vi "Dispose Gabor RefNum.vi"(5 "error in (no error)":errorcluster, 8 "RefNum in":T1) -> (0 "error out":errorcluster)   [LabVIEW 2017, in "SoundVib_Gabor.lvlib"]
doc: "Disposes of the data block referenced by <B>RefNum in</B>."
uses:
  <vilib>/addons/Sound and Vibration/Order Analysis/Gabor Order Tracking/SoundVib_Gabor.lvlib
  <vilib>/addons/Sound and Vibration/Order Analysis/Ref Gabor Order Tracking/GT RefNum.ctl
  <resource>/sndvib.dll
panel:
  # "Dispose Gabor RefNum"
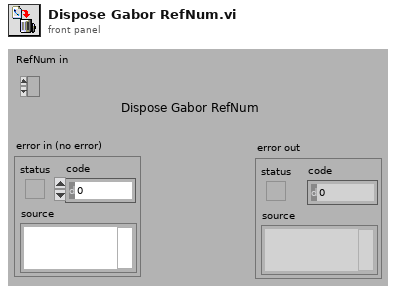
[diagram p1: front panel]
types:
  T1 = typedef "SoundVib_Gabor.lvlib/GT RefNum.ctl" = refnum<k1>
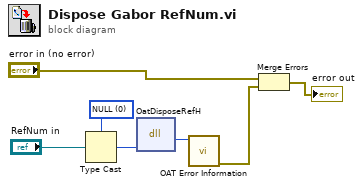
[diagram p0: block diagram]
diagram:
  w4 = u32 0 items=["NULL"]
  n1 = Type Cast(type=w4, x="RefNum in") -> (*(type *) &x=w6:u32)
  n2 = dll-call lib="C:/Program Files (x86)/National Instruments/LabVIEW 2017/resource/sndvib.*" fn="OatDisposeRefH"("Ref In"=w6) -> ("return type"=w7:i32)  [unwired: 4 in, 2 out]
  n3 = call <vilib>:"OAT Error Information.vi"("error code"=w7) -> ("error out"=w1:errorcluster)  [unwired: 6 in]
  n4 = Merge Errors("error in (no error)", w1) -> (→"error out":errorcluster)
